vi "PR Run.vi"   [LabVIEW 2022 SP3, in "BS6006PRPLUS.lvlib"]
doc: "When the status of analog-to-digital converter is disabled, the function would trigger the pulser/Receiver starts to generate the pulse according to the pulse repetition frequency until the PR_Stop() is performed. When the function is performed, the status of analog-to-digital converter is set to be disabled automatically. \n\nextern \"C\" BS6006PRPLUS_API void __cdecl PR_Run();"
uses:
  BS6006PRPLUS.lvlib
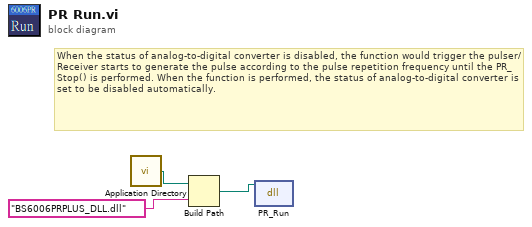
[diagram p0: block diagram]
diagram:
  # "When the status of analog-to-digital converter is disabled, the function would trigger the pulser/Receiver starts to generate the pulse according to the pulse repetition frequency until the PR_Stop() is performed. When the function is performed, the status of analog-to-digital converter is set to be disabled automatically."
  n1 = call <vilib>:"Application Directory.vi"() -> ("Application Directory"=w3:path)
  n2 = Build Path(base path=w3, name or relative path="BS6006PRPLUS_DLL.dll") -> (appended path=w1:path)
  n3 = dll-call lib="E:/Broadsound_Program/PulserReceiver/6006PR PLUS/API/DLL/LabVIEW 15/VIs/BS6006PRPLUS_DLL.dlls" fn="PR_Run"(path in=w1) -> ()  [unwired: 3 in, 2 out]
